vi "UpdateVersiofile.vi"(8 "error in (no error)":errorcluster, 9 "LastVersion":T1, 10 "msg":string, 11 "file (use dialog)":path=path "P:/Departments/Production IT/Software/GVS/BetaTest_NOT_FOR_PRODUCTION/.metadata/release info.txt") -> (0 "error out":errorcluster)   [LabVIEW 2017]
uses:
  <vilib>/AppBuilder/AB_API_Simple/Build Specification Version.ctl
  <vilib>/AppBuilder/AB_API_Simple/NI_App_Builder_API.lvlib
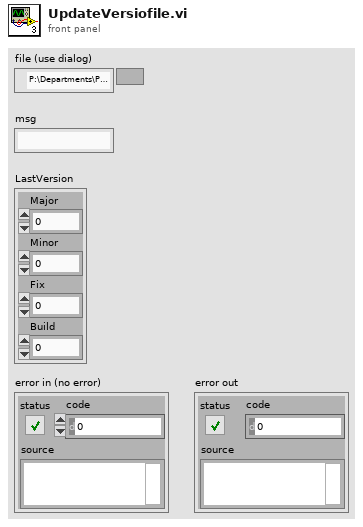
[diagram p1: front panel]
types:
  T1 = typedef "NI_App_Builder_API.lvlib/Build Specification Version.ctl" = cluster{"Major":u16, "Minor":u16, "Fix":u16, "Build":u16}
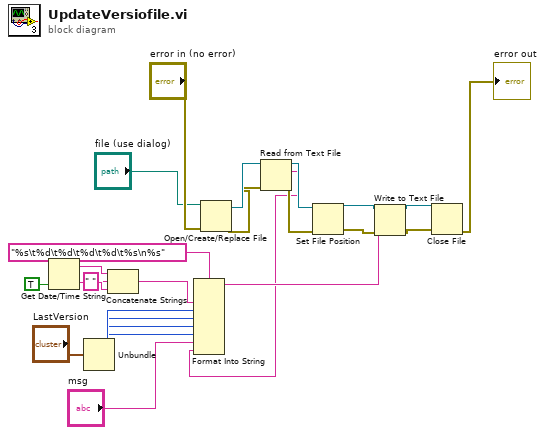
[diagram p0: block diagram]
diagram:
  n1 = Get Date/Time String(want seconds? (F)=TRUE) -> (date string=w17:string, time string=w16:string)  [unwired: 2 in]
  n2 = Unbundle("LastVersion") -> ("Major"=w11:u16, "Minor"=w10:u16, "Fix"=w9:u16, "Build"=w8:u16)
  n3 = Concatenate Strings(w17, " " ("string"), w16) -> (w12:string)
  n4 = Open/Create/Replace File(file path (use dialog)="file (use dialog)", error in="error in (no error)") -> (refnum out=w5:refnum<file>, error out=w4:errorcluster)  [unwired: 4 in, 1 out]
  n5 = Read from Text File(file (use dialog)=w5, error in=w4) -> (refnum out=w3:refnum<file>, text=w1:string, error out=w2:errorcluster)  [unwired: 2 in, 1 out]
  n6 = Format Into String(format string="%s\t%d\t%d\t%d\t%d\t%s\n%s", w12, w11, w10, w9, w8, "msg", w1) -> (resulting string=w6:string)  [unwired: 2 in, 1 out]
  n7 = Set File Position(refnum=w3, error in=w2) -> (refnum out=w20:refnum<file>, error out=w23:errorcluster)  [unwired: 2 in]
  n8 = Write to Text File(file (use dialog)=w20, text=w6, error in=w23) -> (refnum out=w21:refnum<file>, error out=w22:errorcluster)  [unwired: 1 in, 1 out]
  n9 = Close File(refnum=w21, error in=w22) -> (error out=→"error out":errorcluster)  [unwired: 1 out]
